vi "run_tests_with_detailed_report_g-cli.vi"() -> (2 "stdout | stderr":string, 3 "Return Code":i32)   [LabVIEW 2020]
doc: "The module takes in all the Test vi's whose name starts with \"test_\" inside the 'Tests` folder and run it to see if there are any error occuring in the test. Excludes the test mention in `skip_tests.lst`. Finally logs a report on the test results"
uses:
  <vilib>/Wiresmith Technology/G CLI/CLI Class/Output.ctl
  <vilib>/Utility/error.llb/DialogType.ctl
  20ab466a-1420-47d7-bd04-4ec556d045c0.vi
  <vilib>/Utility/error.llb/Error Cluster From Error Code.vi
  <vilib>/Comparison/Equal/Equal Functor/Equal Functor.lvclass
  <vilib>/ErrorRing/Error Ring.xnode
  <vilib>/Wiresmith Technology/G CLI/CLI Class/CLI.lvclass
  Runtime/MeasurementLink Discovery V1/MeasurementLink Discovery V1.lvlib
  Tests.Runtime/Measurement Server/MeasurementServerTests.lvlib
panel:
  out "Custom Parameters":string[](array[string])
  out "Detailed Test Results path":path
  out "Tests Run Time (s)":dbl
  in  "error in":errorcluster
  out "Full Report":string
  out "All Tests Passed":bool
  out "error out":errorcluster
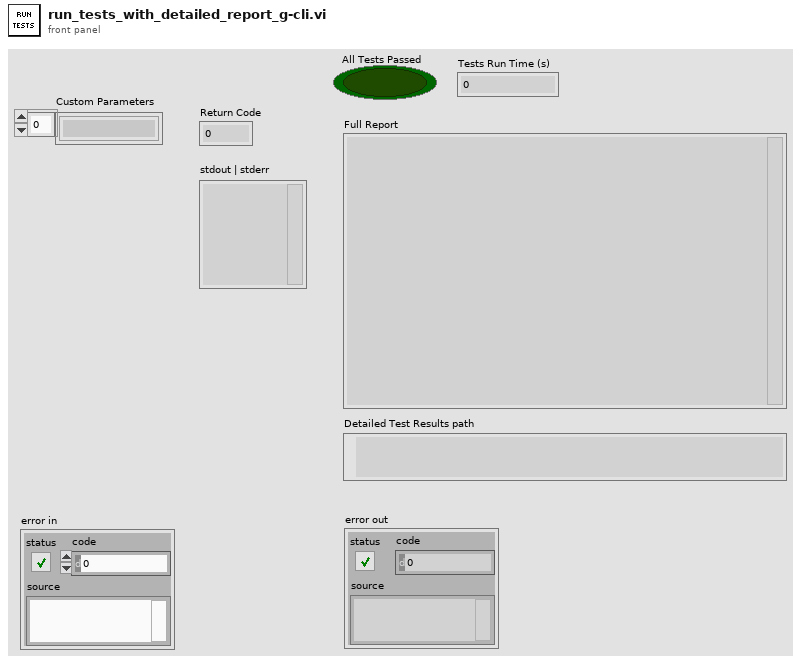
[diagram p1: front panel]
types:
  T1 = typedef "CLI.lvclass/Output.ctl" = enum16{"StdOut", "StdErr"}
  T2 = enum16{"open", "replace", "create", "open or create", "replace or create", "replace or create with confirmation"}
  T3 = typedef "DialogType.ctl" = u16
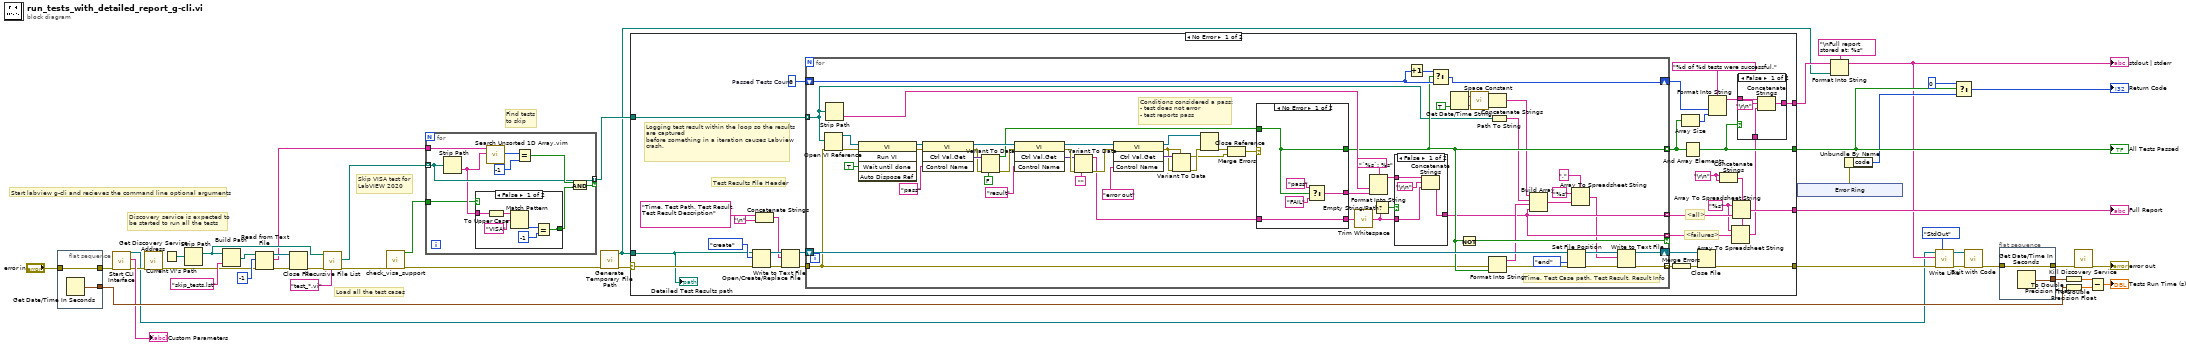
[diagram p0: block diagram]
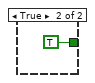
[diagram p2: hidden frame]
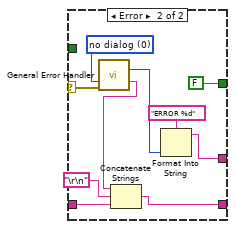
[diagram p5: hidden frame]
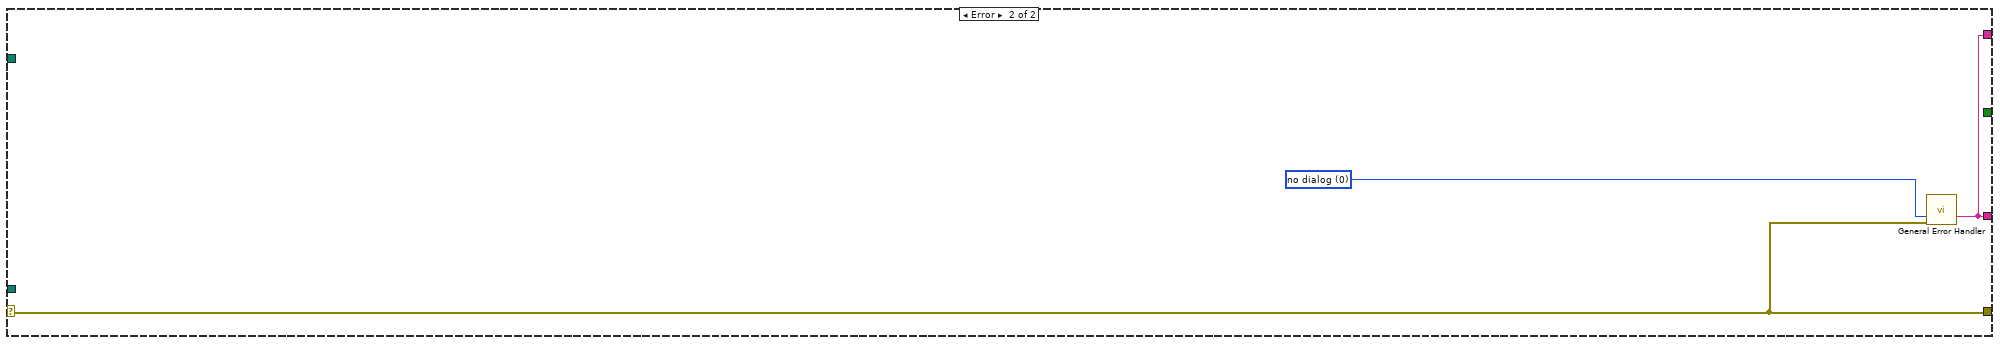
[diagram p6: hidden frame]
diagram:
  # "Discovery service is expected to \nbe started to run all the tests"
  # "Start labview g-cli and recieves the command line optional arguments"
  # "Load all the test cases"
  # "Skip VISA test for LabVIEW 2020"
  # "Find tests\nto skip"
  n1 = flat-sequence {
    tunnel: [w46] -> w21
    tunnel: "error in" -> [w45]
    tunnel: [w45] -> w16
    frame #0 {
      n2 = Get Date/Time In Seconds() -> (seconds since 1Jan1904=w46:timestamp)
    }
  }
  n3 = call <vilib>:"Start CLI Interface.vi"("error in (no error)"=w16) -> ("error out"=w9:errorcluster, "Custom Parameters"=→"Custom Parameters":string[], "CLI out"=w3:refnum<class "CLI.lvclass">)  [unwired: 7 in, 1 out]
  n4 = call "Get Discovery Service Address.vi"("error in"=w9) -> ("error out"=w10:errorcluster)  [unwired: 9 in, 1 out]
  n5 = Current VI's Path() -> (path=w44:path)
  n6 = Strip Path(path=w44) -> (stripped path=w32:path)  [unwired: 1 out]
  n7 = Build Path(base path=w32, name or relative path="skip_tests.lst") -> (appended path=w30:path)
  n8 = Read from Text File(file (use dialog)=w30, count=-1, error in=w10) -> (refnum out=w33:refnum<file>, text=w27:string[], error out=w35:errorcluster)  [unwired: 1 in, 1 out]
  n9 = Close File(refnum=w33, error in=w35) -> (error out=w34:errorcluster)  [unwired: 1 out]
  n10 = call <vilib>:"Recursive File List.vi"("pattern"="test_*.vi", "error in (no error)"=w34, "Folder Path"=w32) -> ("error out"=w24:errorcluster, "All Files in Dir"=w28:path[])  [unwired: 4 in, 3 out]
  n11 = call "check_visa_support.vi"("error in"=w24) -> ("error out"=w6:errorcluster, "visa supported"=w25:bool)  [unwired: 9 in]
  n12 = for {
    tunnel: w28 -> [w50] mode=indexing
    tunnel: w27 -> [w55]
    tunnel: [w50] -> w26 mode=indexing if=w52
    tunnel: w25 -> [w47]
    n13 = Strip Path(path=w50) -> (name=w48:string)  [unwired: 1 out]
    n14 = case shown="False" w47 {
      tunnel: [w56 TRUE] -> w49
      tunnel: w48 -> [w57 _]
      frame False {
        n15 = To Upper Case(1:w57) -> (0:w61:string)
        n16 = Match Pattern(string=w61, regular expression="VISA") -> (offset past match=w60:i32)  [unwired: 1 in, 3 out]
        n17 = Equal?(x=w60, y=-1) -> (x = y?=w56:bool)
      }
      frame True {
      }
    }
    n18 = call "Search Unsorted 1D Array.vim"("element"=w48, "unsorted 1D array"=w55) -> ("index of element"=w54:i32)  [unwired: 9 in]
    n19 = Equal?(x=w54, y=-1) -> (x = y?=w53:bool)
    n20 = And(x=w53, y=w49) -> (x .and. y?=w52:bool)
  }
  n21 = call <vilib>:"Generate Temporary File Path.vi"("error in (no error)"=w6) -> ("error out"=w5:errorcluster, "Unique Temporary File Path"=w4:path)  [unwired: 9 in]
  n22 = case shown="No Error" w5 {
    selector: w5 -> [w64 w180]
    tunnel: w26 -> [w92 _]
    tunnel: [w65 w180] -> w14
    tunnel: [w85 _] -> w40
    tunnel: [w82 w178] -> w41
    tunnel: [w83 w178] -> w8
    tunnel: w4 -> [w63 _]
    frame No Error {
      w89 = 0  # Passed Tests Count
      w78 = "%s" ("format string")
      w91 = "\r\n"
      # "Logging test result within the loop so the results are captured\nbefore something in a iteration causes Labview crash."
      # "Test Results File Header"
      # "<failures>"
      # "<all>"
      n23 = Open/Create/Replace File(file path (use dialog)=w63, error in=w64, operation (0:open)=T2."create") -> (refnum out=w72:refnum<file>, error out=w71:errorcluster)  [unwired: 3 in, 1 out]
      n24 = Concatenate Strings("Time, Test Path, Test Result, Test Result Description" ("text"), "\n") -> (w67:string)
      n25 = Write to Text File(file (use dialog)=w72, text=w67, error in=w71) -> (refnum out=w69:refnum<file>, error out=w70:errorcluster)  [unwired: 1 in, 1 out]
      n26 = for {
        tunnel: w92 -> [w101] mode=indexing
        tunnel: w70 -> [w98]
        tunnel: [w109] -> w87 mode=indexing
        tunnel: [w107] -> w81 mode=indexing
        tunnel: [w107] -> w80 mode=indexing if=w124
        shift-right: [w111] -> w88
        shift-left: w89 -> [w122]
        tunnel: [w118] -> w75 mode=indexing
        shift-right: [w117] -> w76
        shift-left: w69 -> [w110]
        # "Time, Test Case path, Test Result, Result Info"
        # "Conditions considered a pass:\n- test does not error\n- test reports pass"
        n27 = Open VI Reference(vi path=w101, error in (no error)=w98) -> (vi reference=w157:refnum<vi>, error out=w156:errorcluster)  [unwired: 4 in]
        n28 = Strip Path(path=w101) -> (name=w121:string)  [unwired: 1 out]
        n29 = invoke class="VI" method="Run VI"(reference=w157, error in=w156, "Wait until done"=TRUE ("Wait Until Done")) -> (reference out=w154:refnum<vi>, error out=w153:errorcluster)  [unwired: 2 in, 3 out]
        n30 = invoke class="VI" method="Ctrl Val.Get"(reference=w154, error in=w153, "Control Name"="pass") -> (reference out=w143:refnum<vi>, error out=w150:errorcluster, "Get Control Value Variant"=w151:variant)  [unwired: 1 in, 1 out]
        n31 = Variant To Data(error in=w150, type=FALSE, Variant=w151) -> (data=w132:bool, error out=w147:errorcluster)
        n32 = invoke class="VI" method="Ctrl Val.Get"(reference=w143, error in=w147, "Control Name"="result") -> (reference out=w138:refnum<vi>, error out=w148:errorcluster, "Get Control Value Variant"=w145:variant)  [unwired: 1 in, 1 out]
        n33 = Variant To Data(error in=w148, type="", Variant=w145) -> (data=w129:string, error out=w141:errorcluster)
        n34 = invoke class="VI" method="Ctrl Val.Get"(reference=w138, error in=w141, "Control Name"="error out") -> (reference out=w137:refnum<vi>, error out=w139:errorcluster, "Get Control Value Variant"=w142:variant)  [unwired: 1 in, 1 out]
        n35 = Variant To Data(error in=w139, type=w139, Variant=w142) -> (data=w134:errorcluster, error out=w140:errorcluster)
        n36 = Close Reference(reference=w137, error in (no error)=w140) -> (error out=w135:errorcluster)
        n37 = Merge Errors(w135, w134) -> (w133:errorcluster)
        n38 = case shown="No Error" w133 {
          selector: w133 -> [_ w175]
          tunnel: w132 -> [w165 _]
          tunnel: [w164 w172] -> w130
          tunnel: [w165 FALSE] -> w109
          tunnel: w129 -> [w163 w171]
          tunnel: [w163 w170] -> w128
          frame No Error {
            n39 = Select(t="pass" ("Control Name"), s=w165, f="FAIL" ("Control Name")) -> (s? t:f=w164:string)
          }
          frame Error {
            w176 = T3 0 items=["no dialog", "OK message", "continue or stop message", "OK message + warnings", "continue/stop + warnings"] ("type of dialog (OK msg:1)")
            n40 = call <vilib>:"General Error Handler.vi"("type of dialog (OK msg:1)"=w176, "error in (no error)"=w175) -> ("code out"=w174:i32, "message"=w169:string)  [unwired: 9 in, 3 out]
            n41 = Concatenate Strings(w169, "\r\n", w171) -> (w170:string)
            n42 = Format Into String(format string="ERROR %d", w174) -> (resulting string=w172:string)  [unwired: 2 in, 1 out]
          }
        }
        n43 = call <vilib>:"Trim Whitespace.vi"("string"=w128) -> ("trimmed string"=w127:string)  [unwired: 1 in]
        n44 = Format Into String(format string="`%s`: %s" ("Control Name"), w121, w130) -> (resulting string=w125:string)  [unwired: 2 in, 1 out]
        n45 = Empty String/Path?(string/path=w127) -> (empty?=w126:bool)
        n46 = case shown="False" w126 {
          tunnel: w127 -> [w160 _]
          tunnel: w125 -> [w161 w162]
          tunnel: [w159 w162] -> w107
          frame False {
            n47 = Concatenate Strings(w161, "\r\n", w160) -> (w159:string)
          }
          frame True {
          }
        }
        n48 = Increment(x=w122) -> (x+1=w123:i32)
        n49 = Select(t=w123, s=w109, f=w122) -> (s? t:f=w111:i32)
        n50 = Get Date/Time String(want seconds? (F)=TRUE) -> (date string=w114:string, time string=w112:string)  [unwired: 2 in]
        n51 = Not(x=w109) -> (.not. x?=w124:bool)
        n52 = call <vilib>:"Space Constant.vi"() -> ("String"=w113:string)
        n53 = Concatenate Strings(w114, w113, w112) -> (w102:string)
        n54 = Format Into String(error in=w98, w109) -> (resulting string=w108:string, error out=w99:errorcluster)  [unwired: 2 in]
        n55 = Path To String(path=w101) -> (string=w100:string)
        n56 = Build Array(w102, w100, w108, w107) -> (w106:string[])
        n57 = Set File Position(refnum=w110, from (0:start)=enum16{"start", "end", "current"}."end", error in=w99) -> (refnum out=w119:refnum<file>, error out=w120:errorcluster)  [unwired: 1 in]
        n58 = Array To Spreadsheet String(delimiter (Tab)="," ("format string"), array=w106, 3:"%s" ("format string")) -> (spreadsheet string=w103:string)
        n59 = Write to Text File(file (use dialog)=w119, text=w103, error in=w120) -> (refnum out=w117:refnum<file>, error out=w118:errorcluster)  [unwired: 1 in, 1 out]
      }
      n60 = Merge Errors(w75) -> (w74:errorcluster)
      n61 = Array Size(array=w87) -> (size(s)=w86:i32)
      n62 = And Array Elements(Boolean array=w87) -> (logical AND=w85:bool)
      n63 = Close File(refnum=w76, error in=w74) -> (error out=w65:errorcluster)  [unwired: 1 out]
      n64 = Format Into String(format string="%d of %d tests were successful." ("Control Name"), w88, w86) -> (resulting string=w84:string)  [unwired: 2 in, 1 out]
      n65 = Concatenate Strings(w91, w91) -> (w79:string)
      n66 = Array To Spreadsheet String(delimiter (Tab)=w79, array=w80, 3:w78) -> (spreadsheet string=w77:string)
      n67 = Array To Spreadsheet String(delimiter (Tab)=w79, array=w81, 3:w78) -> (spreadsheet string=w82:string)
      n68 = case shown="False" w85 {
        tunnel: w84 -> [w96 w97]
        tunnel: [w93 w97] -> w83
        tunnel: w77 -> [w94 _]
        frame False {
          n69 = Concatenate Strings(w96, "\r\n", w94) -> (w93:string)
        }
        frame True {
        }
      }
      "Detailed Test Results path" <- w63
    }
    frame Error {
      w179 = T3 0 items=["no dialog", "OK message", "continue or stop message", "OK message + warnings", "continue/stop + warnings"] ("type of dialog (OK msg:1)")
      n70 = call <vilib>:"General Error Handler.vi"("type of dialog (OK msg:1)"=w179, "error in (no error)"=w180) -> ("message"=w178:string)  [unwired: 9 in, 4 out]
    }
  }
  "All Tests Passed" <- w40
  "Full Report" <- w41
  n71 = xnode "Error Ring"() -> ("error out"=w37:errorcluster)
  n72 = Format Into String(format string="\nFull report stored at: %s" ("Control Name"), initial string=w8, w4) -> (resulting string=w7:string)  [unwired: 1 in, 1 out]
  "stdout | stderr" <- w7
  n73 = Unbundle By Name(w37) -> ("code"=w36:i32)
  n74 = call <vilib>:"Write Line.vi"("Output (StdOut)"=Output."StdOut", "error in (no error)"=w14, "Text to Write"=w7, "CLI in"=w3) -> ("error out"=w13:errorcluster, "CLI out"=w11:refnum<class "CLI.lvclass">)  [unwired: 6 in]
  n75 = Select(t=0, s=w40, f=w36) -> (s? t:f=→"Return Code":i32)
  n76 = call <vilib>:"Exit with Code.vi"("error in (no error)"=w13, "CLI in"=w11) -> ("error out"=w15:errorcluster)  [unwired: 9 in]
  n77 = flat-sequence {
    tunnel: [w182] -> w22
    tunnel: w15 -> [w181]
    tunnel: [w181] -> w1
    frame #0 {
      n78 = Get Date/Time In Seconds() -> (seconds since 1Jan1904=w182:timestamp)
    }
  }
  n79 = To Double Precision Float(number=w22) -> (double precision float=w19:dbl)
  n80 = To Double Precision Float(number=w21) -> (double precision float=w18:dbl)
  n81 = call "Kill Discovery Service.vi"("error in"=w1) -> ("error out"=→"error out":errorcluster)  [unwired: 10 in]
  n82 = Subtract(x=w19, y=w18) -> (x-y=→"Tests Run Time (s)":dbl)
